vi "Write T.vi"(8 "error in (no error)":errorcluster, 10 "T":dbl[](array[numeric]), 11 "Update Housekeeping in":refnum<class "Update Housekeeping.lvclass">) -> (0 "error out":errorcluster, 3 "Update Housekeeping out":refnum<class "Update Housekeeping.lvclass">)   [LabVIEW 2014, in "eCRDS Library.lvlib" / "Update Housekeeping.lvclass"]
uses:
  Update Housekeeping.lvclass
  Update Housekeeping.lvclass/Update Housekeeping.ctl
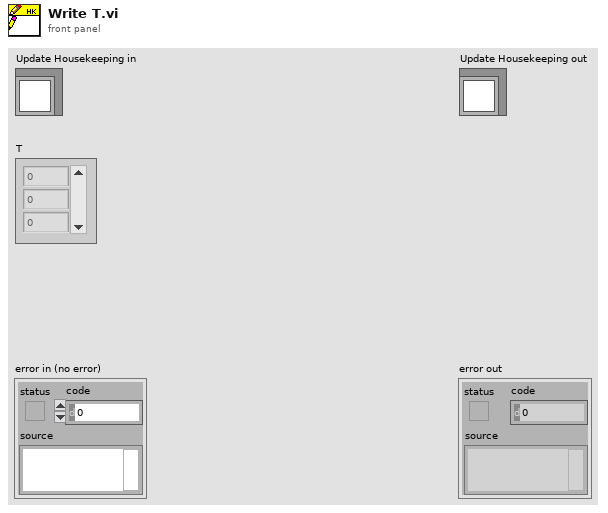
[diagram p1: front panel]
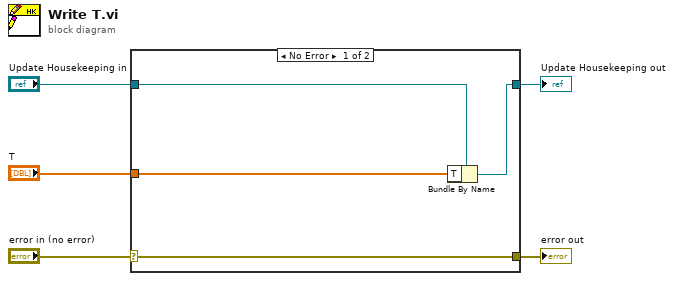
[diagram p0: block diagram]
diagram:
  n1 = case shown="No Error" "error in (no error)" {
    selector: "error in (no error)" -> [w9 w10]
    tunnel: [w9 w10] -> w4
    tunnel: [w7 w11] -> w2
    tunnel: "Update Housekeeping in" -> [w8 w11]
    tunnel: "T" -> [w6 _]
    frame No Error {
      n2 = Bundle By Name(cluster=w8, "T"=w6) -> (w7:refnum<class "Update Housekeeping.lvclass">)
    }
    frame Error {
    }
  }
  "error out" <- w4
  "Update Housekeeping out" <- w2
